vi "File_Writing_U6Instrumentation.vi"(8 "error in (no error)":errorcluster, 10 "Output":T1, 11 "Refnum in":refnum<k34>) -> (0 "error out":errorcluster, 3 "Refnum out":refnum<k34>)   [LabVIEW 2021]
uses:
  Control 1.ctl
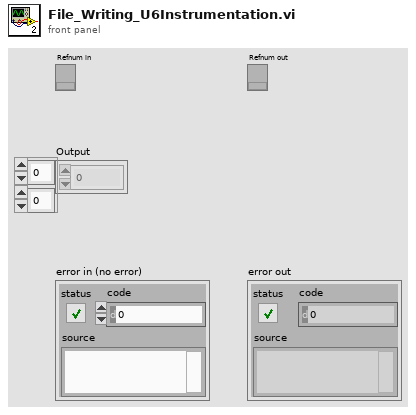
[diagram p1: front panel]
types:
  T1 = typedef "Control 1.ctl" = dbl[][]
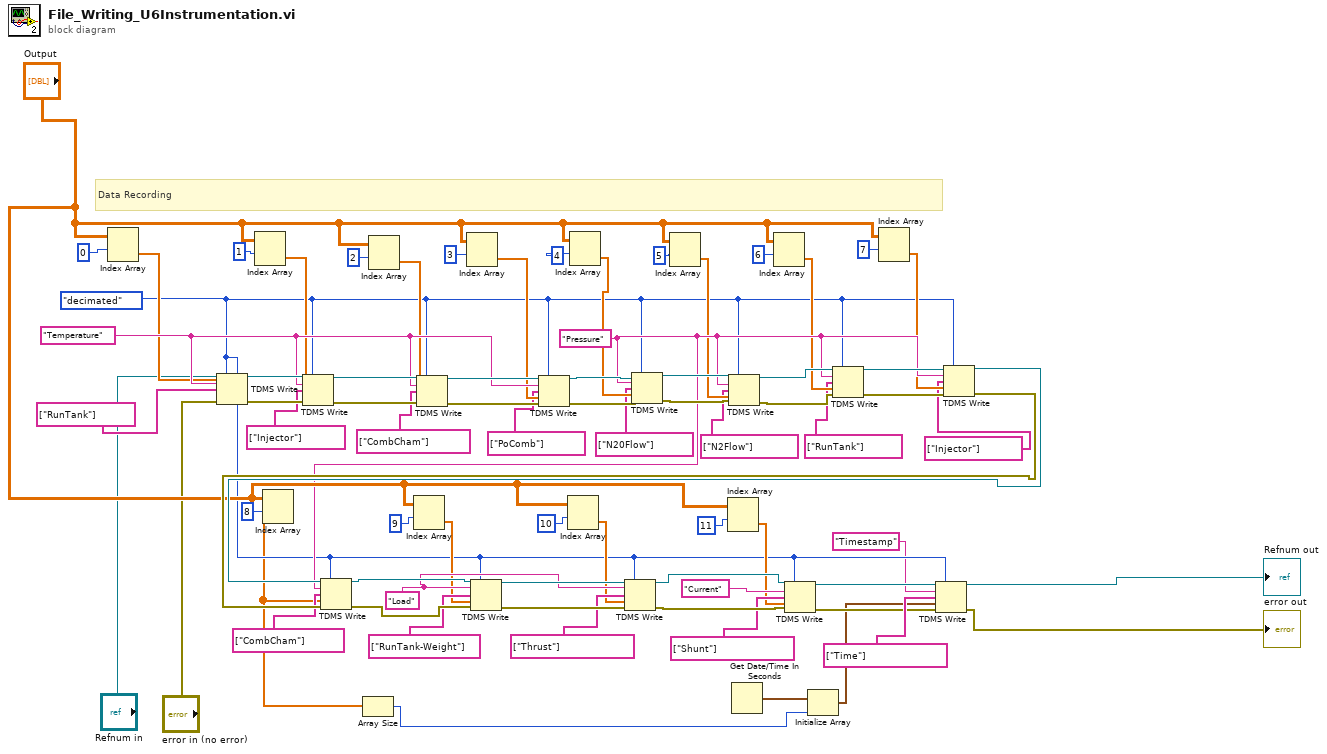
[diagram p0: block diagram]
diagram:
  w48 = "Load" ("group name in (Untitled)")
  w41 = "Pressure" ("group name in (Untitled)")
  w9 = enum16{"decimated", "interleaved"}."decimated" ("data layout (0:decimated)")
  w26 = "Temperature" ("group name in (Untitled)")
  # "Data Recording"
  n1 = Index Array(array="Output", index (row)=0) -> (element=w15:dbl[])  [unwired: 1 in]
  n2 = TDMS Write(0:"Refnum in", 1:w9, 5:w26, 7:string[] ["RunTank"] ("channel name(s) in (Untitled)"), 9:w15, 11:"error in (no error)") -> (4:w65:refnum<k34>, 15:w54:errorcluster)  [unwired: 2 out]
  n3 = Index Array(array="Output", index (row)=1) -> (element=w19:dbl[])  [unwired: 1 in]
  n4 = Index Array(array="Output", index (row)=8) -> (element=w6:dbl[])  [unwired: 1 in]
  n5 = TDMS Write(0:w65, 1:w9, 5:w26, 7:string[] ["Injector"] ("channel name(s) in (Untitled)"), 9:w19, 11:w54) -> (4:w66:refnum<k34>, 15:w55:errorcluster)  [unwired: 2 out]
  n6 = Array Size(array=w6) -> (size(s)=w5:i32)
  n7 = Index Array(array="Output", index (row)=2) -> (element=w21:dbl[])  [unwired: 1 in]
  n8 = Index Array(array="Output", index (row)=9) -> (element=w42:dbl[])  [unwired: 1 in]
  n9 = TDMS Write(0:w66, 1:w9, 5:w26, 7:string[] ["CombCham"] ("channel name(s) in (Untitled)"), 9:w21, 11:w55) -> (4:w67:refnum<k34>, 15:w56:errorcluster)  [unwired: 2 out]
  n10 = Index Array(array="Output", index (row)=3) -> (element=w24:dbl[])  [unwired: 1 in]
  n11 = TDMS Write(0:w67, 1:w9, 5:w26, 7:string[] ["PoComb"] ("channel name(s) in (Untitled)"), 9:w24, 11:w56) -> (4:w68:refnum<k34>, 15:w57:errorcluster)  [unwired: 2 out]
  n12 = Index Array(array="Output", index (row)=10) -> (element=w45:dbl[])  [unwired: 1 in]
  n13 = Index Array(array="Output", index (row)=4) -> (element=w28:dbl[])  [unwired: 1 in]
  n14 = TDMS Write(0:w68, 1:w9, 5:w41, 7:string[] ["N20Flow"] ("channel name(s) in (Untitled)"), 9:w28, 11:w57) -> (4:w69:refnum<k34>, 15:w58:errorcluster)  [unwired: 2 out]
  n15 = Index Array(array="Output", index (row)=5) -> (element=w31:dbl[])  [unwired: 1 in]
  n16 = Index Array(array="Output", index (row)=11) -> (element=w49:dbl[])  [unwired: 1 in]
  n17 = TDMS Write(0:w69, 1:w9, 5:w41, 7:string[] ["N2Flow"] ("channel name(s) in (Untitled)"), 9:w31, 11:w58) -> (4:w70:refnum<k34>, 15:w59:errorcluster)  [unwired: 2 out]
  n18 = Get Date/Time In Seconds() -> (seconds since 1Jan1904=w7:timestamp)
  n19 = Index Array(array="Output", index (row)=6) -> (element=w34:dbl[])  [unwired: 1 in]
  n20 = Initialize Array(w7, w5) -> (w4:timestamp[])
  n21 = TDMS Write(0:w70, 1:w9, 5:w41, 7:string[] ["RunTank"] ("channel name(s) in (Untitled)"), 9:w34, 11:w59) -> (4:w71:refnum<k34>, 15:w60:errorcluster)  [unwired: 2 out]
  n22 = Index Array(array="Output", index (row)=7) -> (element=w37:dbl[])  [unwired: 1 in]
  n23 = TDMS Write(0:w71, 1:w9, 5:w41, 7:string[] ["Injector"] ("channel name(s) in (Untitled)"), 9:w37, 11:w60) -> (4:w72:refnum<k34>, 15:w61:errorcluster)  [unwired: 2 out]
  n24 = TDMS Write(0:w72, 1:w9, 5:w41, 7:string[] ["CombCham"] ("channel name(s) in (Untitled)"), 9:w6, 11:w61) -> (4:w73:refnum<k34>, 15:w62:errorcluster)  [unwired: 2 out]
  n25 = TDMS Write(0:w73, 1:w9, 5:w48, 7:string[] ["RunTank-Weight"] ("channel name(s) in (Untitled)"), 9:w42, 11:w62) -> (4:w74:refnum<k34>, 15:w63:errorcluster)  [unwired: 2 out]
  n26 = TDMS Write(0:w74, 1:w9, 5:w48, 7:string[] ["Thrust"] ("channel name(s) in (Untitled)"), 9:w45, 11:w63) -> (4:w75:refnum<k34>, 15:w64:errorcluster)  [unwired: 2 out]
  n27 = TDMS Write(0:w75, 1:w9, 5:"Current" ("group name in (Untitled)"), 7:string[] ["Shunt"] ("channel name(s) in (Untitled)"), 9:w49, 11:w64) -> (4:w8:refnum<k34>, 15:w10:errorcluster)  [unwired: 2 out]
  n28 = TDMS Write(0:w8, 1:w9, 5:"Timestamp" ("group name in (Untitled)"), 7:string[] ["Time"] ("channel name(s) in (Untitled)"), 9:w4, 11:w10) -> (4:→"Refnum out":refnum<k34>, 15:→"error out":errorcluster)  [unwired: 2 out]
